vi "ArrayToIDToArray.vi"(10 "array in ?":bool, 11 "Array in":u8[](array[numeric])) -> (2 "Array out":u8[](array[numeric]) format="%.0x", 3 "Device ID out":u32)   [LabVIEW 2019]
panel:
  in  "Device ID in":u32
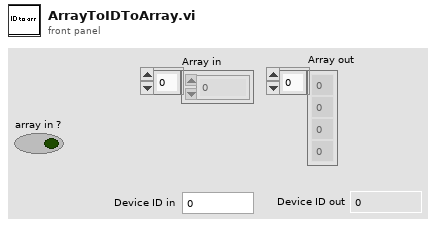
[diagram p1: front panel]
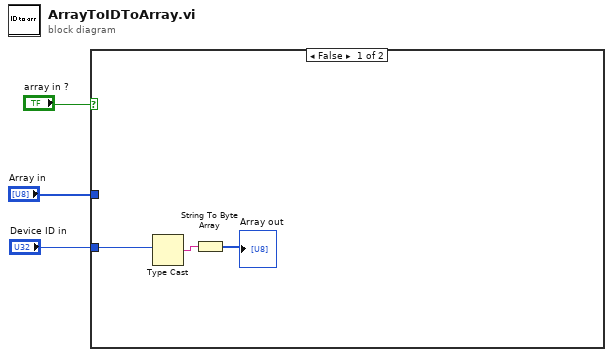
[diagram p0: block diagram]
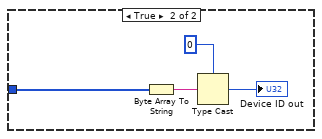
[diagram p2: hidden frame]
diagram:
  n1 = case shown="False" "array in ?" {
    tunnel: "Array in" -> [_ w7]
    tunnel: "Device ID in" -> [w4 _]
    frame False {
      n2 = Type Cast(x=w4) -> (*(type *) &x=w5:string)  [unwired: 1 in]
      n3 = String To Byte Array(string=w5) -> (unsigned byte array=→"Array out":u8[])
    }
    frame True {
      n4 = Byte Array To String(unsigned byte array=w7) -> (string=w9:string)
      n5 = Type Cast(type=u32 0 ("S2"), x=w9) -> (*(type *) &x=→"Device ID out":u32)
    }
  }
